vi "ParseSensorDryVars.vi"(0 "GEA2 Reference In":refnum<k24>, 5 "GEA Inputs":T2={"Source"=228, "Destination"=36} {"Destination" format="%.0x"; "Source" format="%.0x"}, 7 "SnsrDryERD":T3[](array[typedef]) {"ERD Number" format="%.0x"}, 11 "Error In":errorcluster) -> (4 "GEA2 Reference Out":refnum<k24>, 6 "SensorDryVars":T1, 15 "Error out":errorcluster)   [LabVIEW 2016]
uses:
  Q:/Common/DLLs/GEA3/GeaCommunication.dll
  Common/DLLs/GEA3/GeaCommunication.dll
  Common/LabVIEW GEA2 Toolkit/LabVIEW_GEA2_Toolkit.lvlibp/type defs/ERD Read Data In.ctl
  Common/LabVIEW GEA2 Toolkit/LabVIEW_GEA2_Toolkit.lvlibp/type defs/Data Type.ctl
  Common/LabVIEW GEA2 Toolkit/LabVIEW_GEA2_Toolkit.lvlibp/type defs/Source_Destination.ctl
  TyeDefs/SensorDryVars.ctl
  Common/LabVIEW GEA2 Toolkit/LabVIEW_GEA2_Toolkit.lvlibp
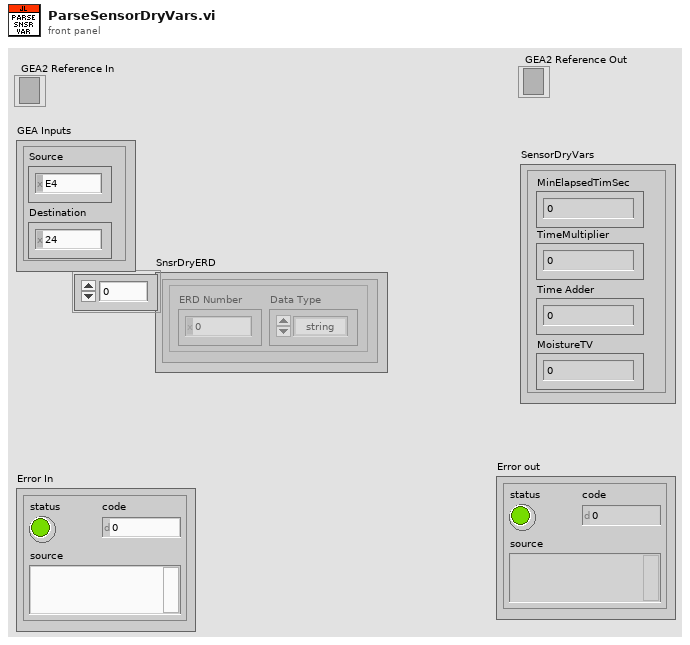
[diagram p1: front panel]
types:
  T1 = typedef "SensorDryVars.ctl" = cluster{"MinElapsedTimSec":u32, "TimeMultiplier":u32, "Time Adder":u32, "MoistureTV":u32}
  T2 = typedef "LabVIEW_GEA2_Toolkit.lvlibp/Source_Destination.ctl" = cluster{"Source":u8, "Destination":u8}
  T3 = typedef "LabVIEW_GEA2_Toolkit.lvlibp/ERD Read Data In.ctl" = cluster{"ERD Number":u16, "Data Type":T4}
  T4 = typedef "LabVIEW_GEA2_Toolkit.lvlibp/Data Type.ctl" = enum16{"string", "boolean", "uint8_t", "uint16_t", "uint32_t", "uint64_t", "int8_t", "int16_t", "int32_t", "int64_t"}
  T5 = typedef "LabVIEW_GEA2_Toolkit.lvlibp/ERD Read Data Out.ctl" = cluster{"ERD Number":u16, "Data":string}
  T6 = cluster{"ERD Data Out[0]":T5, "ERD Data Out[1]":T5, "ERD Data Out[2]":T5, "ERD Data Out[3]":T5, "ERD Data Out[4]":T5, "ERD Data Out[5]":T5, "ERD Data Out[6]":T5, "ERD Data Out[7]":T5, "ERD Data Out[8]":T5}
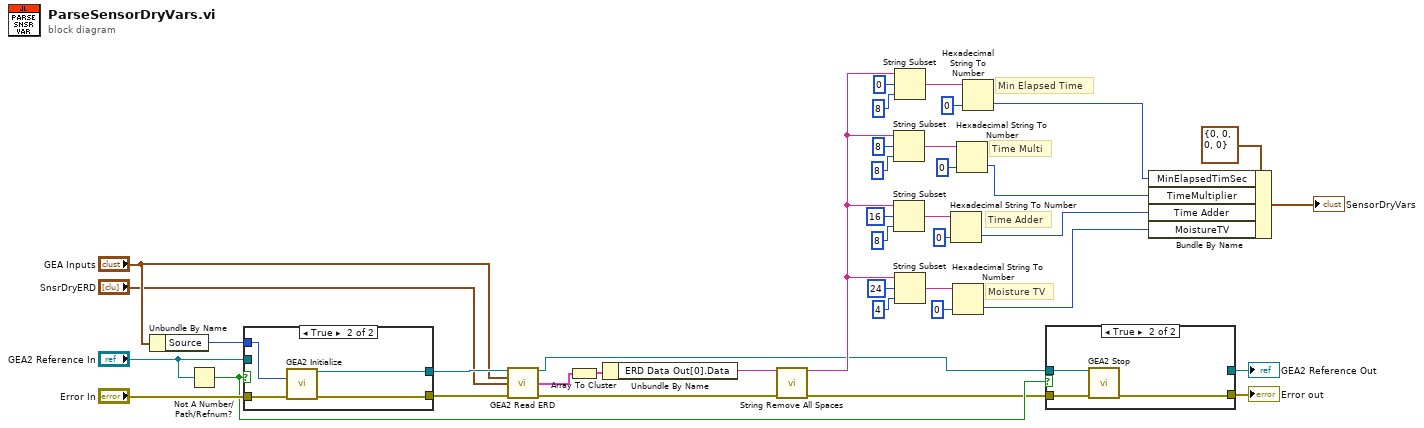
[diagram p0: block diagram]
diagram:
  # "Moisture TV"
  # "Time Adder"
  # "Time Multi"
  # "Min Elapsed Time"
  n1 = Unbundle By Name("GEA Inputs") -> ("Source"=w34:u8)
  n2 = Not A Number/Path/Refnum?(number/path/refnum="GEA2 Reference In") -> (NaN/Path/Refnum?=w6:bool)
  n3 = case shown="True" w6 {
    tunnel: "GEA2 Reference In" -> [w41 _]
    tunnel: [w41 w45] -> w37
    tunnel: "Error In" -> [w40 w44]
    tunnel: [w40 w43] -> w36
    tunnel: w34 -> [_ w42]
    frame False {
    }
    frame True {
      n4 = call "GEA2 Initialize.vi"("Source Address"=w42, "error in"=w44) -> ("GEA2 Reference Out"=w45:refnum<k24>, "error out"=w43:errorcluster)  [unwired: 11 in, 1 out]
    }
  }
  n5 = call "GEA2 Read ERD.vi"("GEA2 Reference In"=w37, "GEA Inputs"="GEA Inputs", "Read ERD List"="SnsrDryERD", "Error In"=w36) -> ("GEA2 Reference Out"=w4:refnum<k24>, "ERD Data Out"=w33:T5[], "Error Out"=w17:errorcluster)  [unwired: 8 in, 1 out]
  n6 = Array To Cluster(array=w33) -> (cluster=w32:T6)
  n7 = Unbundle By Name(w32) -> ("ERD Data Out[0].Data"=w31:string)
  n8 = call "String Remove All Spaces.vi"("Input String"=w31, "error in (no error)"=w17) -> ("Spaces Removed"=w22:string, "error out"=w5:errorcluster)  [unwired: 12 in]
  n9 = String Subset(string=w22, offset (0)=u8 8, length (rest)=8 ("length (rest)")) -> (substring=w18:string)
  n10 = String Subset(string=w22, offset (0)=u8 16, length (rest)=8 ("length (rest)")) -> (substring=w19:string)
  n11 = String Subset(string=w22, offset (0)=u8 0, length (rest)=8 ("length (rest)")) -> (substring=w21:string)
  n12 = String Subset(string=w22, offset (0)=u8 24, length (rest)=4 ("length (rest)")) -> (substring=w20:string)
  n13 = Hexadecimal String To Number(string=w19, default (0uL)=u32 0 ("default (0 U32)")) -> (number=w8:u32)  [unwired: 1 in, 1 out]
  n14 = Hexadecimal String To Number(string=w20, default (0uL)=u32 0 ("default (0 U32)")) -> (number=w7:u32)  [unwired: 1 in, 1 out]
  n15 = Hexadecimal String To Number(string=w18, default (0uL)=u32 0 ("default (0 U32)")) -> (number=w9:u32)  [unwired: 1 in, 1 out]
  n16 = Hexadecimal String To Number(string=w21, default (0uL)=u32 0 ("default (0 U32)")) -> (number=w10:u32)  [unwired: 1 in, 1 out]
  n17 = case shown="True" w6 {
    tunnel: w4 -> [w47 w48]
    tunnel: [w47 _] -> w3
    tunnel: w5 -> [w46 w50]
    tunnel: [w46 w49] -> w2
    frame False {
    }
    frame True {
      n18 = call "GEA2 Stop.vi"("GEA2 Reference In"=w48, "Error In"=w50) -> ("Error Out"=w49:errorcluster)  [unwired: 13 in]
    }
  }
  "GEA2 Reference Out" <- w3
  "Error out" <- w2
  n19 = Bundle By Name(cluster=T1 {"MinElapsedTimSec"=0, "TimeMultiplier"=0, "Time Adder"=0, "MoistureTV"=0} ("SensorDryVars"), "MinElapsedTimSec"=w10, "TimeMultiplier"=w9, "Time Adder"=w8, "MoistureTV"=w7) -> (→"SensorDryVars":T1)
